vi "Experiment 8.vi"() -> ()   [LabVIEW 2026]
doc: "Experiment 8"
panel:
  out "No. Of Iterations Executed - Loop 2":i32
  out "Output - Loop 2":dbl[](array[numeric]) format="%.3f"
  out "No. Of Iterations Executed - Loop 1":i32
  out "Output - Loop 1":dbl[](array[numeric]) format="%.3f"
  out "Stop VI?":bool
  # "Experiment 8"
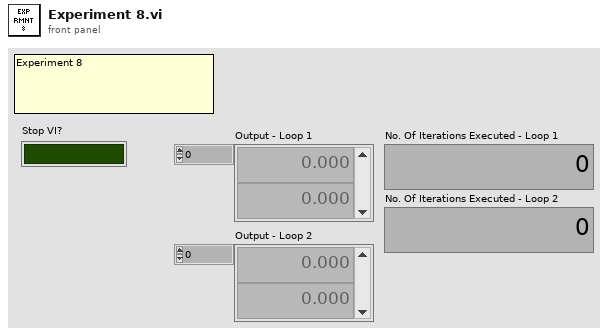
[diagram p1: front panel]
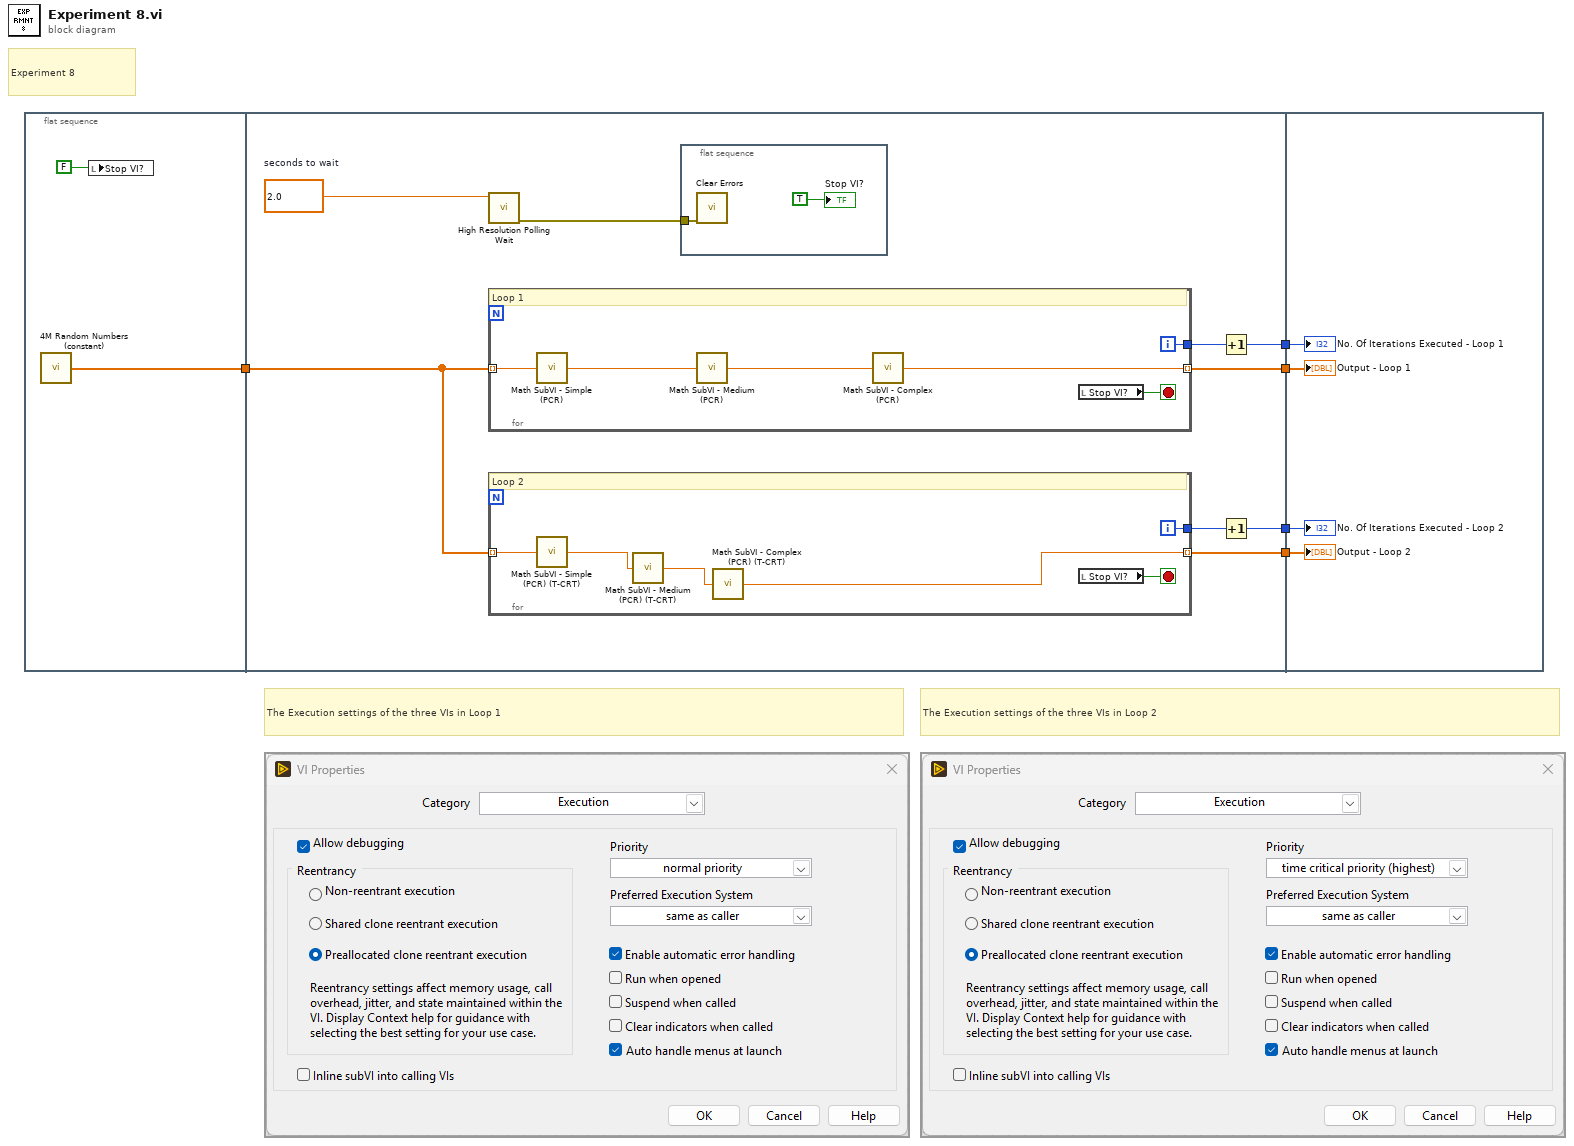
[diagram p0: block diagram]
diagram:
  # "The Execution settings of the three VIs in Loop 2"
  # "The Execution settings of the three VIs in Loop 1"
  # "Experiment 8"
  n1 = flat-sequence {
    tunnel: [w6] -> w1
    tunnel: [w14] -> w5
    tunnel: [w12] -> w4
    tunnel: [w11] -> w3
    tunnel: [w9] -> w2
    tunnel: w1 -> [w8]
    tunnel: w5 -> [w34]
    tunnel: w4 -> [w32]
    tunnel: w3 -> [w31]
    tunnel: w2 -> [w33]
    frame #0 {
      n2 = call "4M Random Numbers (constant).vi"() -> ("4M Random Numbers"=w6:dbl[])
      n3 = local write "Stop VI?"(FALSE) -> ()
    }
    frame #1 {
      w16 = 2.0  # seconds to wait
      n4 = call <vilib>:"High Resolution Polling Wait.vi"("seconds to wait"=w16) -> ("error out"=w15:errorcluster)  [unwired: 10 in]
      n5 = for {
        tunnel: w8 -> [w28] mode=indexing
        tunnel: [w25] -> w14 mode=indexing
        tunnel: [w26] -> w13
        i -> [w26]
        stop <- w27 stop-if-true
        # "Loop 1"
        n6 = call "Math SubVI - Simple (PCR).vi"("Input"=w28) -> ("Output"=w23:dbl)
        n7 = call "Math SubVI - Medium (PCR).vi"("Input"=w23) -> ("Output"=w24:dbl)
        n8 = call "Math SubVI - Complex (PCR).vi"("Input"=w24) -> ("Output"=w25:dbl)
        n9 = local read "Stop VI?"() -> (w27:bool)
      }
      n10 = for {
        tunnel: w8 -> [w20] mode=indexing
        tunnel: [w19] -> w9 mode=indexing
        tunnel: [w21] -> w10
        i -> [w21]
        stop <- w22 stop-if-true
        # "Loop 2"
        n11 = call "Math SubVI - Simple (PCR) (T-CRT).vi"("Input"=w20) -> ("Output"=w17:dbl)
        n12 = call "Math SubVI - Medium (PCR) (T-CRT).vi"("Input"=w17) -> ("Output"=w18:dbl)
        n13 = call "Math SubVI - Complex (PCR) (T-CRT).vi"("Input"=w18) -> ("Output"=w19:dbl)
        n14 = local read "Stop VI?"() -> (w22:bool)
      }
      n15 = flat-sequence {
        tunnel: w15 -> [w29]
        frame #0 {
          n16 = call <vilib>:"Clear Errors.vi"("error in (no error)"=w29) -> ()  [unwired: 5 in, 2 out]
          "Stop VI?" <- TRUE
        }
      }
      n17 = Increment(x=w13) -> (x+1=w12:i32)
      n18 = Increment(x=w10) -> (x+1=w11:i32)
    }
    frame #2 {
      "No. Of Iterations Executed - Loop 1" <- w32
      "Output - Loop 1" <- w34
      "No. Of Iterations Executed - Loop 2" <- w31
      "Output - Loop 2" <- w33
    }
  }
